vi "set msg (sub to event).vi"(8 "error in (no error)":errorcluster, 9 "State":string(combo), 10 "MSG":string(combo), 11 "Domino Laser module Class in":refnum<class "Domino Laser module Class.lvclass">) -> (0 "error out":errorcluster, 3 "Domino Laser module Class out":refnum<class "Domino Laser module Class.lvclass">)   [LabVIEW 2015, in "Domino LM.lvlib" / "Domino Laser module Class.lvclass"]
uses:
  CTRLS/Domino Laser module Class.lvclass
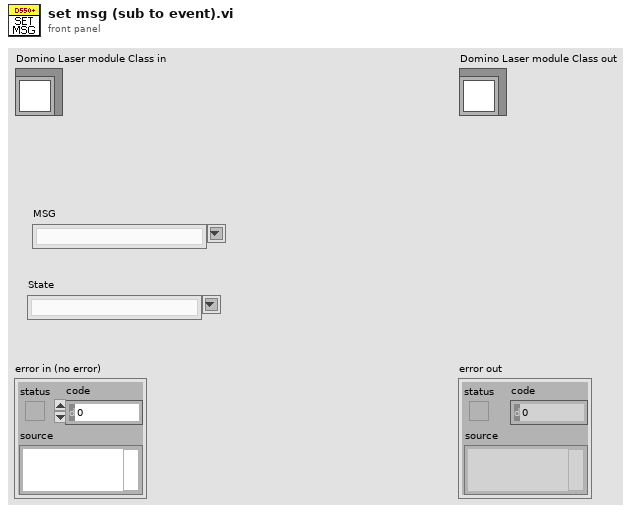
[diagram p1: front panel]
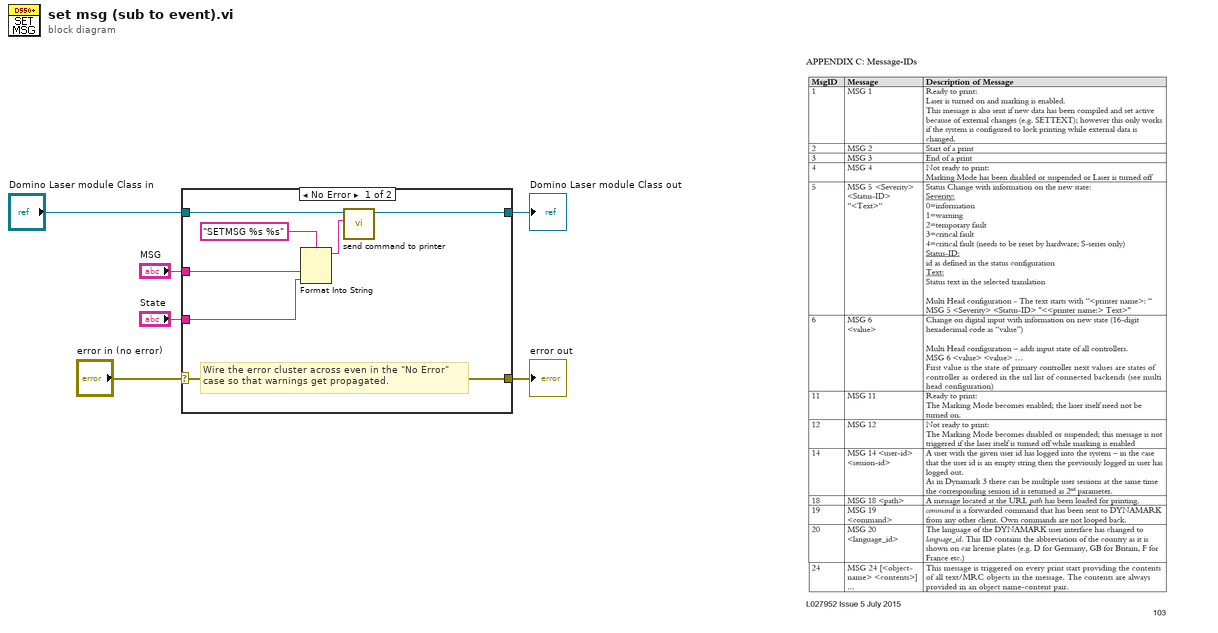
[diagram p0: block diagram]
diagram:
  n1 = case shown="No Error" "error in (no error)" {
    selector: "error in (no error)" -> [w13 w15]
    tunnel: [w13 w15] -> w5
    tunnel: [w11 w14] -> w3
    tunnel: "Domino Laser module Class in" -> [w12 w14]
    tunnel: "MSG" -> [w9 _]
    tunnel: "State" -> [w8 _]
    frame No Error {
      # "Wire the error cluster across even in the \"No Error\"\ncase so that warnings get propagated."
      n2 = Format Into String(format string="SETMSG %s %s", w9, w8) -> (resulting string=w7:string)  [unwired: 2 in, 1 out]
      n3 = call "send command to printer.vi"("command to be sent"=w7, "Domino Laser module Class in"=w12) -> ("Domino Laser module Class out"=w11:refnum<class "Domino Laser module Class.lvclass">)  [unwired: 6 in, 3 out]
    }
    frame Error {
    }
  }
  "error out" <- w5
  "Domino Laser module Class out" <- w3
